vi "Stop Work.vi"(6 "Controller name":string, 8 "error in (no error)":errorcluster, 9 "Reply":bool=TRUE, 10 "Reply to":refnum<class "Stop Response Msg.lvclass">, 11 "Spectrum Recorder in":refnum<class "Spectrum Recorder.lvclass">) -> (0 "error out":errorcluster, 3 "Spectrum Recorder out":refnum<class "Spectrum Recorder.lvclass">)   [LabVIEW 2024, in "Spectrum Recorder.lvclass"]
uses:
  Spectrum Recorder.lvclass
  Spectrum Recorder.lvclass/Spectrum Recorder.ctl
  NHMFL_Core/Libraries/Instruments/Instrument Driver/Worker State.ctl
  Controllers/Process Controller Messages/Stop Response Msg/Stop Response Msg.lvclass
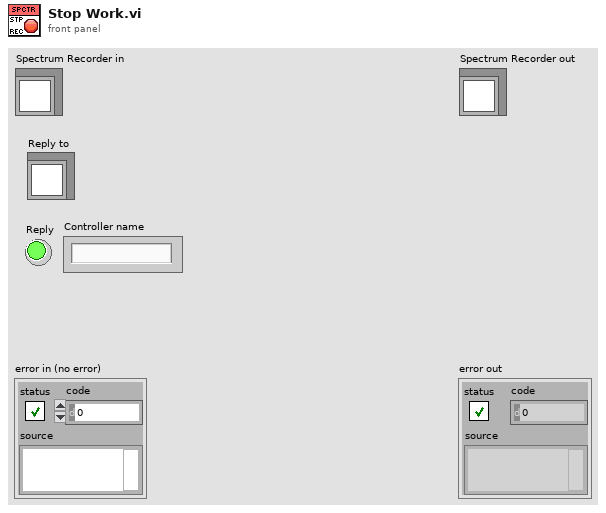
[diagram p1: front panel]
types:
  T1 = typedef "Worker State.ctl" = enum16{"Idle", "Starting", "Working", "Stopping"}
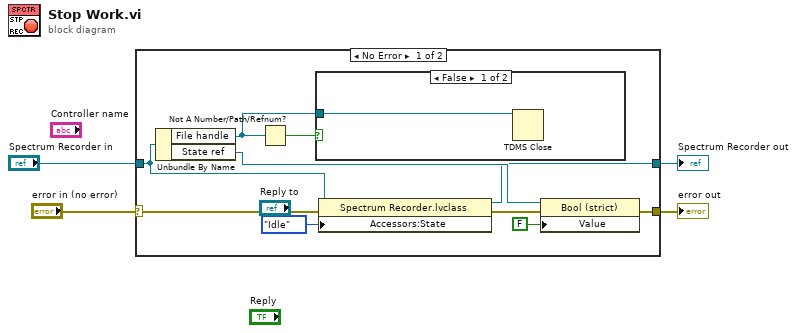
[diagram p0: block diagram]
diagram:
  n1 = case shown="No Error" "error in (no error)" {
    selector: "error in (no error)" -> [w7 w17]
    tunnel: [w11 w17] -> w3
    tunnel: [w8 w16] -> w1
    tunnel: "Spectrum Recorder in" -> [w14 w16]
    frame No Error {
      n2 = Unbundle By Name(w14) -> ("File handle"=w12:refnum<k34>, "State ref"=w9:refnum<vi>)
      n3 = Not A Number/Path/Refnum?(number/path/refnum=w12) -> (NaN/Path/Refnum?=w13:bool)
      n4 = case shown="False" w13 {
        tunnel: w12 -> [w15 _]
        frame False {
          n5 = TDMS Close(11:w15) -> ()  [unwired: 1 in, 2 out]
        }
        frame True {
        }
      }
      n6 = property class="Spectrum Recorder.lvclass"(reference=w14, error in=w7, "Accessors:State"=Worker_State."Idle" ("State")) -> (reference out=w8:refnum<class "Spectrum Recorder.lvclass">, error out=w6:errorcluster)
      n7 = property class="Bool (strict)"(reference=w9, error in=w6, "Value"=FALSE) -> (error out=w11:errorcluster)  [unwired: 1 out]
    }
    frame Error {
    }
  }
  "error out" <- w3
  "Spectrum Recorder out" <- w1
